vi "TwSetFloatAttributeInH5.vi"(0 "error in (no error)":errorcluster, 1 "filename":string, 2 "location":string, 3 "name":string, 4 "attribute":sgl) -> (5 "error out":errorcluster)   [LabVIEW 2009]
uses:
  TwH5Dll.dll
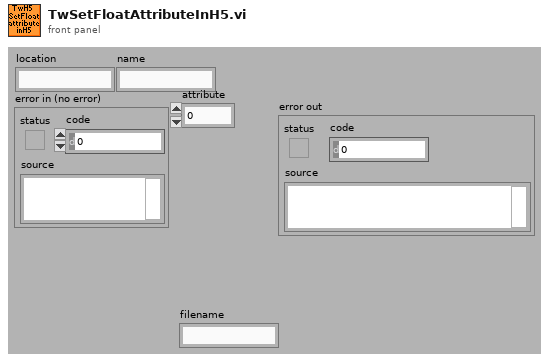
[diagram p1: front panel]
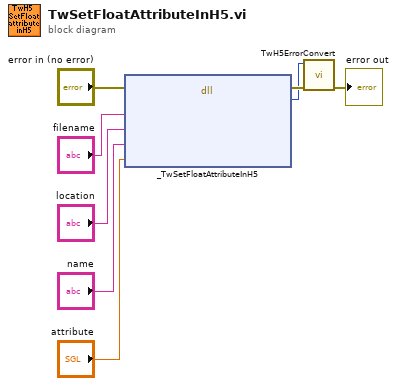
[diagram p0: block diagram]
diagram:
  n1 = dll-call lib="C:/src/85_TofDaq_current/DllWrappers/LabView/TwH5Dll/TwH5Dll.dll" fn="_TwSetFloatAttributeInH5"(error in="error in (no error)", "filename"="filename", "location"="location", "name"="name", "attribute"="attribute") -> (error out=w7:errorcluster, "TwRetVal"=w6:i32)  [unwired: 6 in, 1 out]
  n2 = call "TwH5ErrorConvert.vi"("error in (no error)"=w7, "error code"=w6) -> ("error out"=→"error out":errorcluster)  [unwired: 9 out]
